vi "Bus Interface.vi"(0 "rx core":refnum<class "niUSRP Rx Core v1 FPGA.lvclass">, 1 "abort":bool, 5 "instruction":T2, 9 "input valid":bool) -> (6 "response":T1, 10 "done":bool, 14 "ready for input":bool)   [LabVIEW 2025, in "niUSRP Rx Core v1 FPGA.lvclass"]
uses:
  niUSRP Rx Core v1 FPGA.lvclass
  <instrlib>/_niInstr/Instruction Framework/v1/FPGA/Interfaces/Address Space/Address Space Instruction.ctl
  <instrlib>/_niInstr/Instruction Framework/v1/FPGA/Typedefs/Response.ctl
  niUSRP Rx Core v1 FPGA.lvclass/niUSRP Rx Core v1 FPGA.ctl
  <vilib>/rvi/DataTransferAndStorage/Container/Common/niFpgaContainerExecOnDevCompGetState.vi
  <vilib>/rvi/Emulation/niFpgaEmulationIsFPGAContextNoSignature.vi
  <vilib>/rvi/DataTransferAndStorage/Container/Common/niFpgaContainerGetUniqueNameForEmu.vi
  <vilib>/rvi/Memory/Memory_Emulation/niFpgaMemoryEmulationCacheClearOnFirstRun.vi
  <vilib>/rvi/Memory/Memory_Emulation/nirvimemoryEmulationManagerCache_MakeExclusive.vi
  <vilib>/rvi/Memory/Memory_Emulation/niFpgaMemoryEmulationValidateCache.vi
  <vilib>/rvi/Memory/Memory_Emulation/nirvimemoryEmulationManagerCache_InsertValue.vi
  <vilib>/Utility/error.llb/Clear Errors.vi
  <vilib>/rvi/Memory/Memory_Emulation/nirvimemoryEmulationManagerCache_ReleaseExclusive.vi
  <vilib>/rvi/Memory/Memory_Emulation/nirvimemoryEmulationManagerCache_GetValue.vi
  <vilib>/rvi/Memory/Memory_Emulation/nirvimemoryEmulationManagerCache_SetValue.vi
  <vilib>/rvi/Emulation/niFpgaProcessEmulError.vi
  <vilib>/rvi/Emulation/niFpgaSctlEmulationGetInTimedLoop.vi
  <vilib>/rvi/DataTransferAndStorage/Container/XNode/niFpgaContainer.xnode
  <vilib>/rvi/DataTransferAndStorage/Register/Emulation/niFpgaRegisterEmulationRefIn.vi
  <instrlib>/_niInstr/Instruction Framework/v1/FPGA/Typedefs/niInstr Instruction Framework v1 FPGA.lvlib
  <instrlib>/_niInstr/Instruction Framework/v1/FPGA/Interfaces/Address Space/Address Space.lvclass
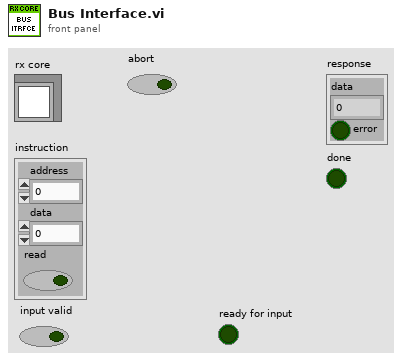
[diagram p1: front panel]
types:
  T1 = typedef "niInstr Instruction Framework v1 FPGA.lvlib/Response.ctl" = cluster{"data":u64, "error":bool}
  T2 = typedef "niInstr Instruction Framework Interfaces v1 FPGA.lvlib/Address Space.lvclass/Address Space Instruction.ctl" = cluster{"address":u32, "data":u64, "read":bool}
  T3 = typedef "niUSRP Rx Core v1 FPGA.lvclass/Regs.ctl" = cluster{"enable":refnum<k21>, "reset":refnum<k21>, "channel no.":u8, "sample clock domain":refnum<k21>, "i in resource":refnum<k21>, "q in resource":refnum<k21>, "Number of Chs":u8, "debug":refnum<k21>, "Loopback FIFO":refnum<k21>}
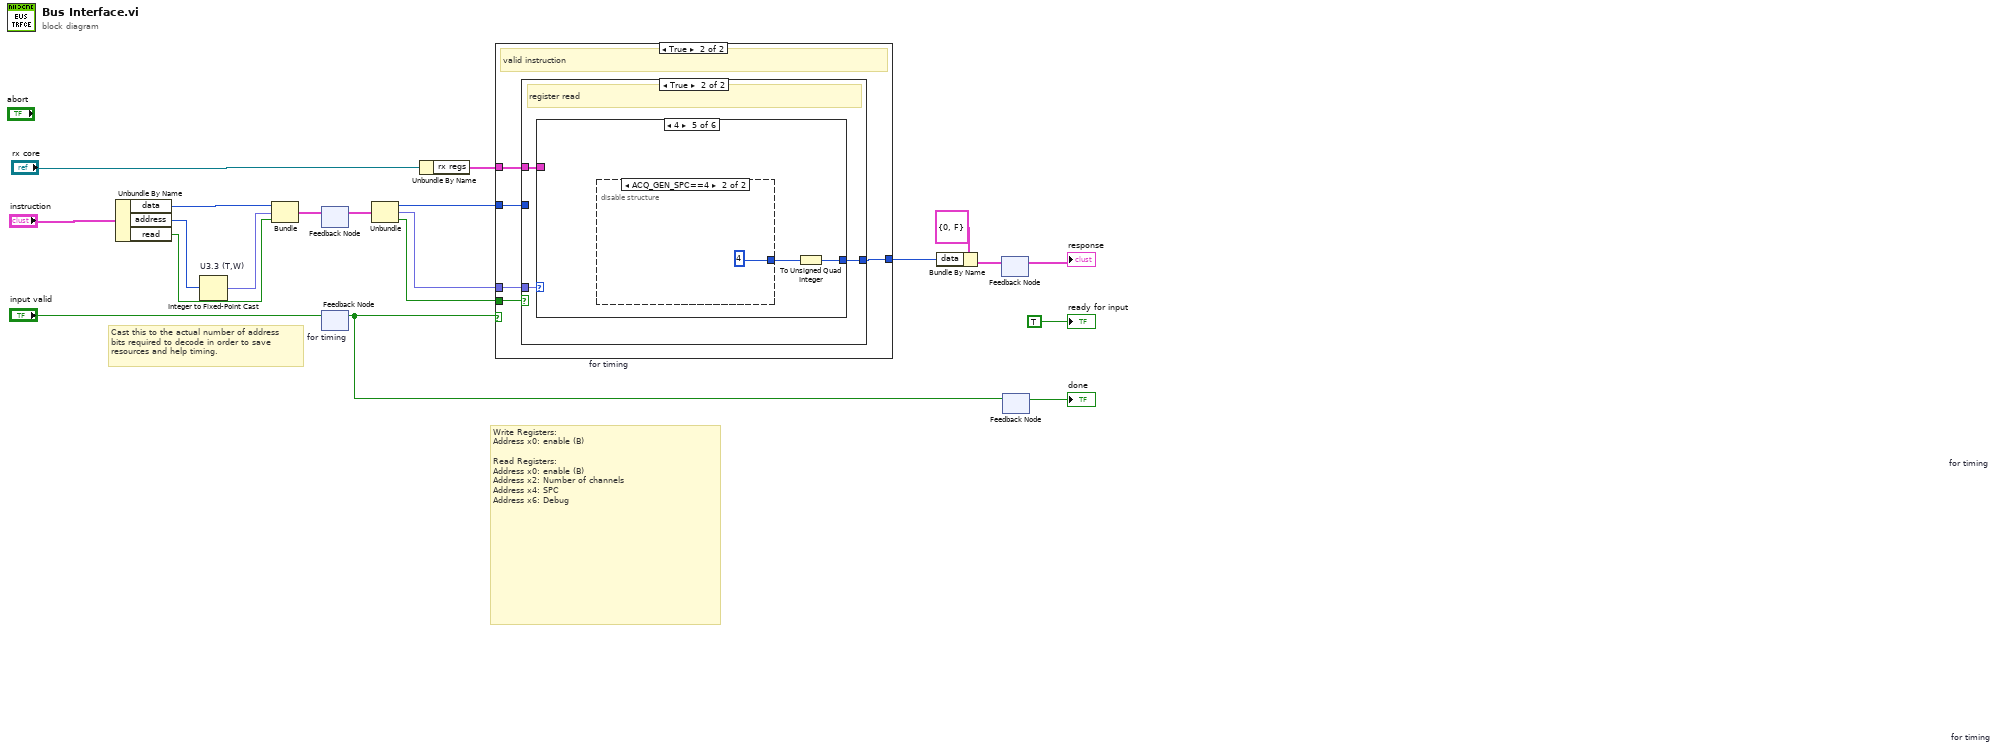
[diagram p0: block diagram]
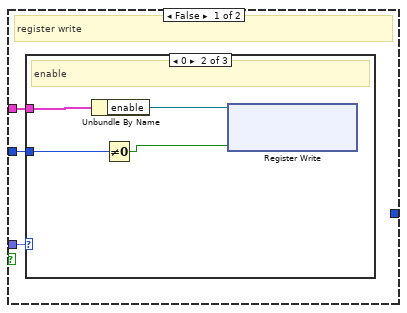
[diagram p3: hidden frame]
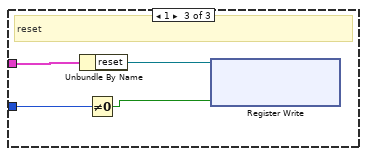
[diagram p5: hidden frame]
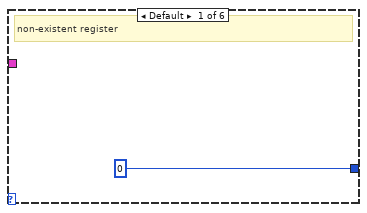
[diagram p6: hidden frame]
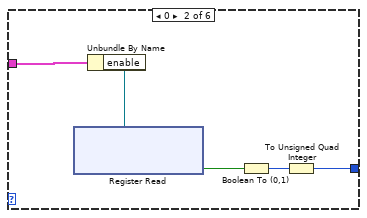
[diagram p7: hidden frame]
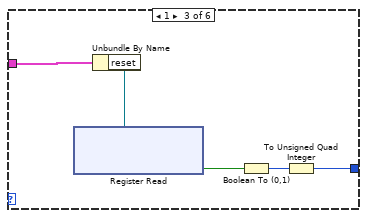
[diagram p8: hidden frame]
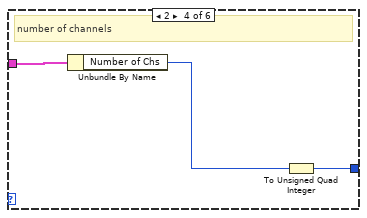
[diagram p9: hidden frame]
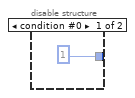
[diagram p10: hidden frame]
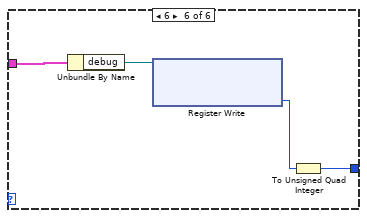
[diagram p11: hidden frame]
diagram:
  # "Write Registers:\nAddress x0: enable (B)\n\nRead Registers:\nAddress x0: enable (B)\nAddress x2: Number of channels\nAddress x4: SPC\nAddress x6: Debug"
  # "Cast this to the actual number of address\nbits required to decode in order to save\nresources and help timing."
  n1 = Unbundle By Name("instruction") -> ("data"=w17:u64, "address"=w20:u32, "read"=w15:bool)
  n2 = Integer to Fixed-Point Cast "U3.3 (T,W)"(integer=w20) -> (fixed-point=w16:fxp<+,3,3>)  [unwired: 1 in]
  n3 = Bundle("data"=w17, w16, "read"=w15) -> (w19:cluster{"data":u64, fxp<+,3,3>, "read":bool})  [unwired: 1 in]
  n4 = feedback #1 "for timing"() -> (w18:cluster{"data":u64, fxp<+,3,3>, "read":bool})  [unwired: 1 in]
  n5 = feedback-in #1(w19) -> ()
  n6 = feedback #2 "for timing"() -> (w1:bool)  [unwired: 1 in]
  n7 = feedback-in #2("input valid") -> ()
  n8 = Unbundle(w18) -> ("data"=w8:u64, w9:fxp<+,3,3>, "read"=w10:bool)
  n9 = Unbundle By Name("rx core") -> ("rx regs"=w11:T3)
  n10 = case shown="True" w1 {
    tunnel: w11 -> [_ w25]
    tunnel: w10 -> [_ w24]
    tunnel: w9 -> [_ w23]
    tunnel: w8 -> [_ w22]
    tunnel: [_ w21] -> w7
    frame False {
      # "invalid instruction"
    }
    frame True {
      # "valid instruction"
      n11 = case shown="True" w24 {
        tunnel: w23 -> [w28 w39]
        tunnel: [_ w38] -> w21
        tunnel: w22 -> [w27 _]
        tunnel: w25 -> [w26 w37]
        frame False {
          # "register write"
          n12 = case shown="0" w28 {
            tunnel: w27 -> [_ w30 w34]
            tunnel: w26 -> [_ w31 w35]
            frame Default {
              # "non-existent register"
            }
            frame 0 {
              # "enable"
              n13 = Unbundle By Name(w31) -> ("enable"=w32:refnum<k21>)
              n14 = Not Equal To 0?(x=w30) -> (x != 0?=w29:bool)
              n15 = xnode ("Register Write")("Data"=w29, "Register In"=w32) -> ()  [unwired: 1 out]
            }
            frame 1 {
              # "reset"
              n16 = Unbundle By Name(w35) -> ("reset"=w36:refnum<k21>)
              n17 = Not Equal To 0?(x=w34) -> (x != 0?=w33:bool)
              n18 = xnode ("Register Write")("Data"=w33, "Register In"=w36) -> ()  [unwired: 1 out]
            }
          }
        }
        frame True {
          # "register read"
          n19 = case shown="4" w39 {
            tunnel: [u64 0 w45 w50 w53 w54 w58] -> w38
            tunnel: w37 -> [_ w43 w48 w52 _ w61]
            frame Default {
              # "non-existent register"
            }
            frame 0 {
              n20 = Unbundle By Name(w43) -> ("enable"=w44:refnum<k21>)
              n21 = xnode ("Register Read")("Register In"=w44) -> ("Data"=w42:bool)  [unwired: 1 out]
              n22 = Boolean To (0,1)(Boolean=w42) -> (0, 1=w41:i16)
              n23 = To Unsigned Quad Integer(1:w41) -> (0:w45:u64)
            }
            frame 1 {
              n24 = Unbundle By Name(w48) -> ("reset"=w49:refnum<k21>)
              n25 = xnode ("Register Read")("Register In"=w49) -> ("Data"=w47:bool)  [unwired: 1 out]
              n26 = Boolean To (0,1)(Boolean=w47) -> (0, 1=w46:i16)
              n27 = To Unsigned Quad Integer(1:w46) -> (0:w50:u64)
            }
            frame 2 {
              # "number of channels"
              n28 = Unbundle By Name(w52) -> ("Number of Chs"=w51:u8)
              n29 = To Unsigned Quad Integer(1:w51) -> (0:w53:u64)
            }
            frame 4 {
              n30 = disable-structure shown="ACQ_GEN_SPC==4" {
                disable-tunnel: [u8 1 ("Number of Chs") u8 4 ("Number of Chs")] -> w55
                frame condition #0 {
                }
                frame condition #1 (active) {
                }
              }
              n31 = To Unsigned Quad Integer(1:w55) -> (0:w54:u64)
            }
            frame 6 {
              n32 = Unbundle By Name(w61) -> ("debug"=w60:refnum<k21>)
              n33 = xnode "Register Write"("Register In"=w60) -> ("Data"=w59:u16)  [unwired: 1 out]
              n34 = To Unsigned Quad Integer(1:w59) -> (0:w58:u64)
            }
          }
        }
      }
    }
  }
  n35 = Bundle By Name(cluster=T1 {"data"=0, "error"=FALSE} ("response"), "data"=w7) -> (w4:T1)
  n36 = feedback #3 "for timing"() -> (→"response":T1)  [unwired: 1 in]
  n37 = feedback-in #3(w4) -> ()
  n38 = feedback #4 "for timing"() -> (→"done":bool)  [unwired: 1 in]
  n39 = feedback-in #4(w1) -> ()
  "ready for input" <- TRUE ("ready for input")
